vi "MGCC_IsdCon_main.vi"   [LabVIEW 2016]
doc: "-----------------------------------------------------------------------------------------------------------------------\nCopyright <2019> <The University of Tennessee at Knoxville and the University of Tennessee Research Foundation>\nThis software is released under BSD-3 \nhttps://opensource.org/licenses/BSD-3-Clause \nAdditional license options available at https://utrf.tennessee.edu/industry/sample-agreements/\n-----------------------------------------------------------------------------------------------------------------------"
uses:
  Finite State Machine/Sub-VIs/MGCC_FntStaMach_gobal.vi
  MGCC_IsdCon_global1.vi
  <vilib>/imath/engines/lvmath2/RunTimeEngine/BuiltInFunctions/size/NIMS_I32=size(GM,I32).vi
  <instcachedir>/0/NIMS_I32=size(GM,I32)_122058B1B3294FAEA5DC209B92B394E4.lvgen/NIMS_I32=size(GM,I32)_122058B1B3294FAEA5DC209B92B394E4_004.vi
  <vilib>/imathl/engines/lvmath/Functions/Error Handling/Create Error.vi
  <vilib>/imath/engines/lvmath2/RunTimeEngine/CommandStatement/MC_CommandStatement_break.vi
  <vilib>/imath/engines/lvmath2/RunTimeEngine/IndexRead/NIMS M(S,S).vi
  <instcachedir>/0/NIMS M(S,S)_AC51E74150A542F7991B9634C66F3096.lvgen/NIMS M(S,S)_AC51E74150A542F7991B9634C66F3096_000.vi
  <vilib>/imath/engines/lvmath2/RunTimeEngine/IndexReplace/NIMS M(S,$)=M.vi
  <instcachedir>/0/NIMS M(S,$)=M_47BFD2E070824516B94BE47F5466D205.lvgen/NIMS M(S,$)=M_47BFD2E070824516B94BE47F5466D205_000.vi
  <vilib>/imath/engines/lvmath2/RunTimeEngine/CommandStatement/NIMS_CommandStatement_MaskErr.vi
  <vilib>/imath/engines/lvmath2/RunTimeEngine/BuiltInFunctions/zeros/NIMS_V=zeros(I32,I32).vi
  <vilib>/imath/engines/lvmath2/RunTimeEngine/ErrorHandling/NIMS_Create Error From Enums.vi
  <vilib>/imath/engines/lvmath2/RunTimeEngine/RangeToken/NIMS_Range_R2 - Float.vi
  <instcachedir>/0/NIMS_Range_R2 - Float_590A1087448447AEB7F770FC082D3801.lvgen/NIMS_Range_R2 - Float_590A1087448447AEB7F770FC082D3801_000.vi
  <vilib>/imath/engines/lvmath2/RunTimeSupport/NIMS_Error if Not Equal.vi
  <instcachedir>/0/NIMS_Error if Not Equal_43252A79AD05436189442EC0C5E5AB8A.lvgen/NIMS_Error if Not Equal_43252A79AD05436189442EC0C5E5AB8A_000.vi
  <vilib>/imath/engines/lvmath2/RunTimeEngine/BuiltInFunctions/size/NIMS_I32=size(GCol,I32).vi
  <instcachedir>/0/NIMS_I32=size(GCol,I32)_3BEAC9C04C22472CB193ADA08E7FE41C.lvgen/NIMS_I32=size(GCol,I32)_3BEAC9C04C22472CB193ADA08E7FE41C_000.vi
  <vilib>/imath/engines/lvmath2/RunTimeEngine/RangeToken/NIMS_Range_R2 - Integer.vi
  <instcachedir>/0/NIMS_Range_R2 - Integer_89B873E74E6E489885E44F751DD9C6BF.lvgen/NIMS_Range_R2 - Integer_89B873E74E6E489885E44F751DD9C6BF_000.vi
  <vilib>/imath/engines/lvmath2/RunTimeEngine/IndexRead/NIMS V(S).vi
  <instcachedir>/0/NIMS V(S)_0488751826AF41519A22953C041130DC.lvgen/NIMS V(S)_0488751826AF41519A22953C041130DC_002.vi
  <vilib>/imath/engines/lvmath2/RunTimeEngine/IndexReplace/NIMS V(S)=S.vi
  <instcachedir>/0/NIMS V(S)=S_57E16554CB8B4B90AAB163894F717546.lvgen/NIMS V(S)=S_57E16554CB8B4B90AAB163894F717546_003.vi
  <vilib>/imath/engines/lvmath2/RunTimeEngine/IndexReplace/NIMS M($,S)=S.vi
  <instcachedir>/0/NIMS M($,S)=S_865F3DAD07AE4A3E845B544A0C6081CA.lvgen/NIMS M($,S)=S_865F3DAD07AE4A3E845B544A0C6081CA_000.vi
  <instcachedir>/0/NIMS M(S,S)_AC51E74150A542F7991B9634C66F3096.lvgen/NIMS M(S,S)_AC51E74150A542F7991B9634C66F3096_002.vi
  <vilib>/imath/engines/lvmath2/RunTimeEngine/IndexReplace/NIMS M(S,S)=S.vi
  <instcachedir>/0/NIMS M(S,S)=S_98E40400474E4398B113AE20298B4F82.lvgen/NIMS M(S,S)=S_98E40400474E4398B113AE20298B4F82_000.vi
  <vilib>/imath/engines/lvmath2/RunTimeEngine/IndexRead/NIMS M($,S).vi
  <instcachedir>/0/NIMS M($,S)_3E5749BBB62E49528D4765A77F1F6D98.lvgen/NIMS M($,S)_3E5749BBB62E49528D4765A77F1F6D98_000.vi
  <vilib>/imath/engines/lvmath2/RunTimeEngine/NodeEndStatement/NIMS_NodeEndStatement_Output.vi
  <instcachedir>/0/NIMS_NodeEndStatement_Output_53EC0D466D134D7ABD903AC30B43404B.lvgen/NIMS_NodeEndStatement_Output_53EC0D466D134D7ABD903AC30B43404B_005.vi
  <vilib>/imath/engines/lvmath2/RunTimeEngine/ErrorHandling/NIMS_Finalize Error.vi
  Communication/Global communication output.vi
  Communication/Global communication.vi
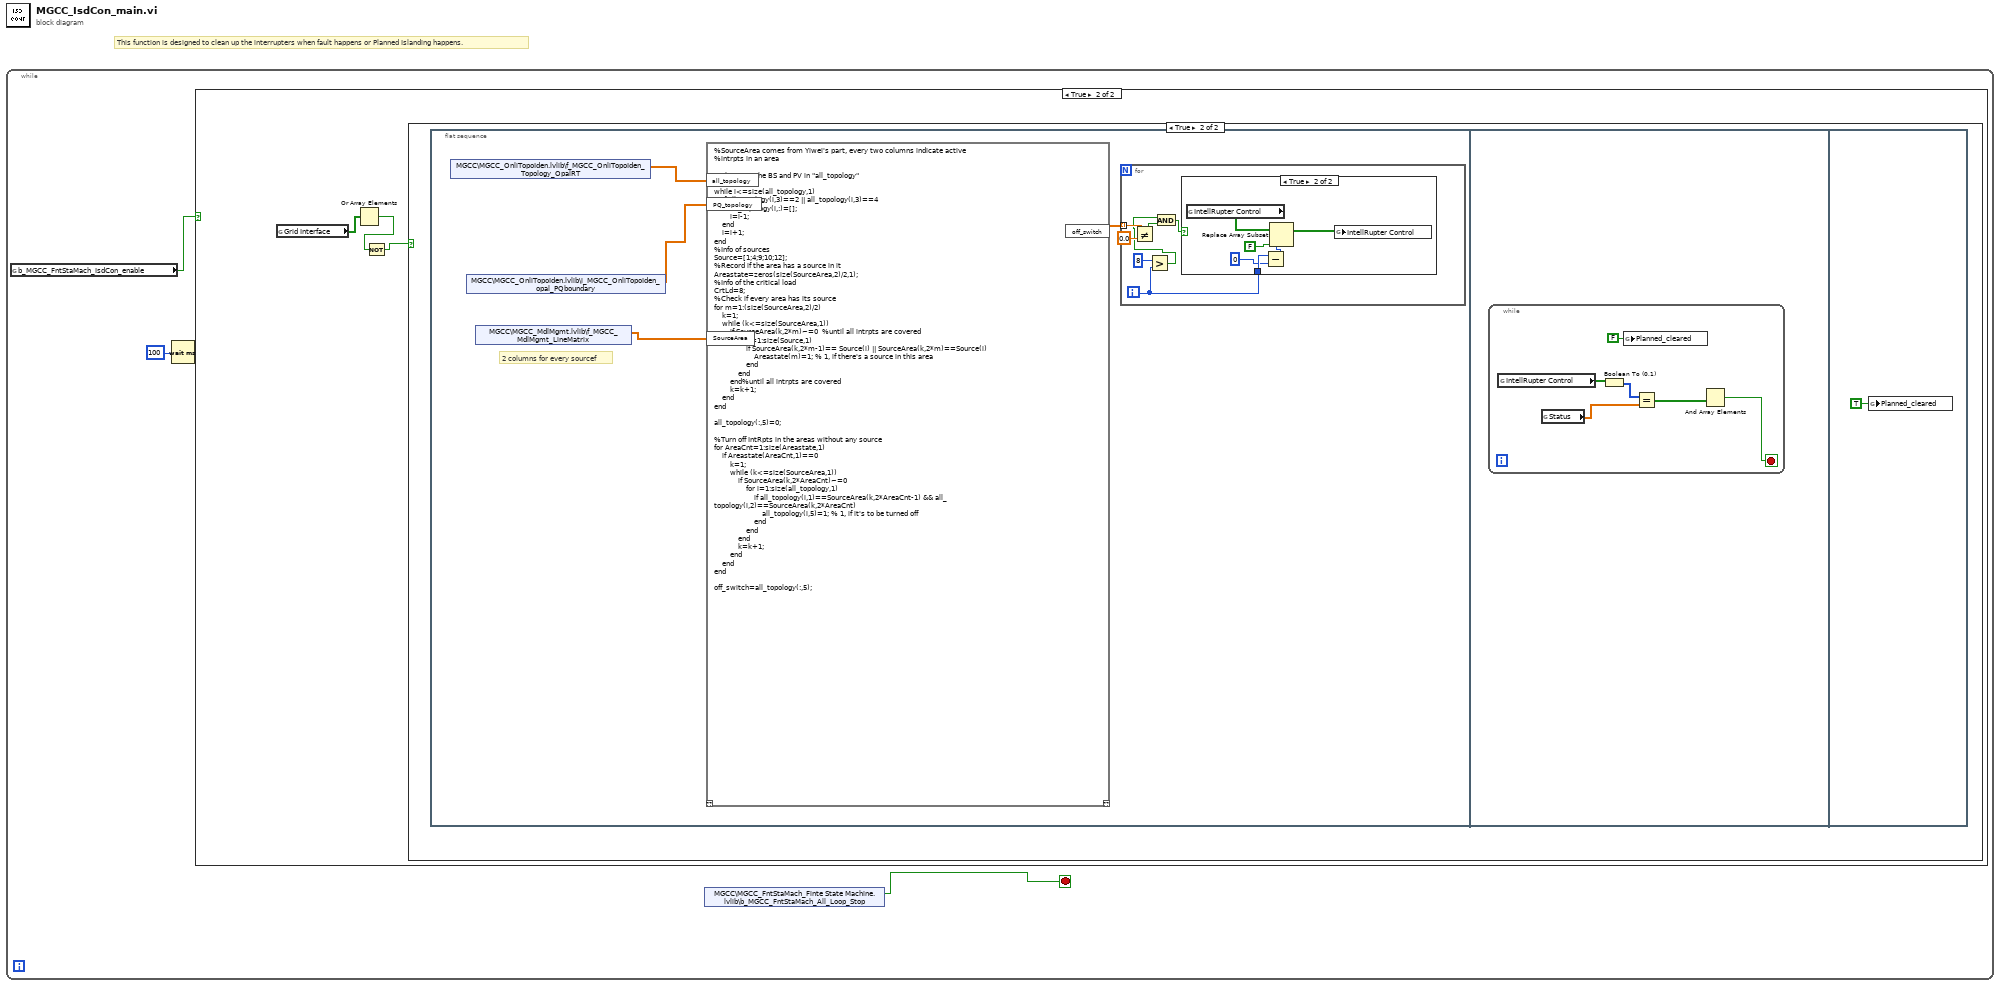
[diagram p0: block diagram]
diagram:
  # "This function is designed to clean up the interrupters when fault happens or Planned Islanding happens."
  n1 = while {
    stop <- w2 stop-if-true
    n2 = global read "MGCC_FntStaMach_gobal.vi" "b_MGCC_FntStaMach_IsdCon_enable"() -> (w1:bool)
    n3 = Wait (ms)(milliseconds to wait=u32 100) -> ()  [unwired: 1 out]
    n4 = case shown="True" w1 {
      frame False {
      }
      frame True {
        n5 = global read "MGCC_IsdCon_global1.vi" "Grid Interface"() -> (w4:bool[])
        n6 = Or Array Elements(Boolean array=w4) -> (logical OR=w6:bool)
        n7 = Not(x=w6) -> (.not. x?=w5:bool)
        n8 = case shown="True" w5 {
          frame False {
          }
          frame True {
            n9 = flat-sequence {
              frame #0 {
                # "2 columns for every sourcef"
                n10 = shared-variable "MGCC\\MGCC_OnliTopoIden.lvlib\\f_MGCC_OnliTopoIden_Topology_OpalRT"() -> (w10:dbl[][])  [unwired: 1 in, 1 out]
                n11 = shared-variable "MGCC\\MGCC_OnliTopoIden.lvlib\\i_MGCC_OnliTopoIden_opal_PQboundary"() -> (w9:dbl[][])  [unwired: 1 in, 1 out]
                n12 = shared-variable "MGCC\\MGCC_MdlMgmt.lvlib\\f_MGCC_MdlMgmt_LineMatrix"() -> (w7:dbl[][])  [unwired: 1 in, 1 out]
                n13 = mathscript code="%SourceArea comes from Yiwei's part, every two columns indicate active\n%intrpts in an area\n\n%Eliminate the BS and PV in \"all_topology\"\ni=1;\nwhile i<=size(all_topology,1)\n    if all_topology(i,3)==2 || all_topology(i,3)==4\n        all_topology(i,:)=[];\n        i=i-1;\n    end\n    i=i+1;\nend\n%Info of sources\nSource=[1;4;9;10;12];\n%Record if the area has a source in it\nAreastate=zeros(size(SourceArea,2)/2,1);\n%Info of the critical load\nCrtLd=8;\n%Check if every area has its source\nfor m=1:(size(SourceArea,2)/2)\n    k=1;\n    while (k<=size(SourceArea,1))\n        if SourceArea(k,2*m)~=0  %until all intrpts are covered\n            for i=1:size(Source,1)\n                if SourceArea(k,2*m-1)== Source(i) || SourceArea(k,2*m)==Source(i)\n                    Areastate(m)=1; % 1, if there's a source in this area\n                end\n            end\n        end%until all intrpts are covered\n        k=k+1;\n    end\nend\n\nall_topology(:,5)=0;\n\n%Turn off IntRpts in the areas without any source\nfor AreaCnt=1:size(Areastate,1)\n    if Areastate(AreaCnt,1)==0\n        k=1;\n        while (k<=size(SourceArea,1))\n            if SourceArea(k,2*AreaCnt)~=0\n                for i=1:size(all_topology,1)\n                    if all_topology(i,1)==SourceArea(k,2*AreaCnt-1) && all_topology(i,2)==SourceArea(k,2*AreaCnt)\n                        all_topology(i,5)=1; % 1, if it's to be turned off\n                    end\n                end\n            end\n            k=k+1;\n        end\n    end\nend\n\noff_switch=all_topology(:,5);"("all_topology"=w10, "PQ_topology"=w9, "SourceArea"=w7) -> ("off_switch"=w8:dbl[])  [unwired: 1 in, 1 out]
                n14 = for {
                  tunnel: w8 -> [w17] mode=indexing
                  i -> [w11]
                  n15 = Not Equal?(x=w17, y=0.0) -> (x != y?=w15:bool)
                  n16 = Greater?(x=8, y=w11) -> (0:w13:bool)
                  n17 = And(x=w13, y=w15) -> (x .and. y?=w14:bool)
                  n18 = case shown="True" w14 {
                    tunnel: w11 -> [_ w20]
                    frame False {
                    }
                    frame True {
                      n19 = global read "Global communication output.vi" "IntellRupter Control"() -> (w23:bool[])
                      n20 = Subtract(x=w20, y=0) -> (x-y=w18:i32)
                      n21 = Replace Array Subset(array=w23, new element=FALSE ("new element/subarray"), index=w18) -> (w22:bool[])
                      n22 = global write "Global communication output.vi" "IntellRupter Control"(w22) -> ()
                    }
                  }
                }
              }
              frame #1 {
                n23 = while {
                  stop <- w929 stop-if-true
                  n24 = global read "Global communication output.vi" "IntellRupter Control"() -> (w933:bool[])
                  n25 = global read "Global communication.vi" "Status"() -> (w932:dbl[])
                  n26 = Boolean To (0,1)(Boolean=w933) -> (0, 1=w931:i16[])
                  n27 = global write "MGCC_IsdCon_global1.vi" "Planned_cleared"(FALSE ("Planned_cleared")) -> ()
                  n28 = Equal?(x=w931, y=w932) -> (x = y?=w930:bool[])
                  n29 = And Array Elements(Boolean array=w930) -> (logical AND=w929:bool)
                }
              }
              frame #2 {
                n30 = global write "MGCC_IsdCon_global1.vi" "Planned_cleared"(TRUE ("Planned_cleared")) -> ()
              }
            }
          }
        }
      }
    }
    n31 = shared-variable "MGCC\\MGCC_FntStaMach_Finte State Machine.lvlib\\b_MGCC_FntStaMach_All_Loop_Stop"() -> (w2:bool)  [unwired: 1 in, 1 out]
  }
